vi "Scripting_GetSubVISourcesDrains.vi"(8 "error in (no error)":errorcluster, 11 "SubVIIn":refnum<vi>) -> (0 "error out":errorcluster, 1 "DrainsSources":T1(array[cluster]), 2 "SourceDrains":T2(array[cluster]), 3 "SubVIOut":refnum<vi>)   [LabVIEW 2016]
panel:
  in  "DeleteWiresToSorcesAndDrains(True)":bool=TRUE
  in  "IgnoreCornerTerminals(True)":bool=TRUE
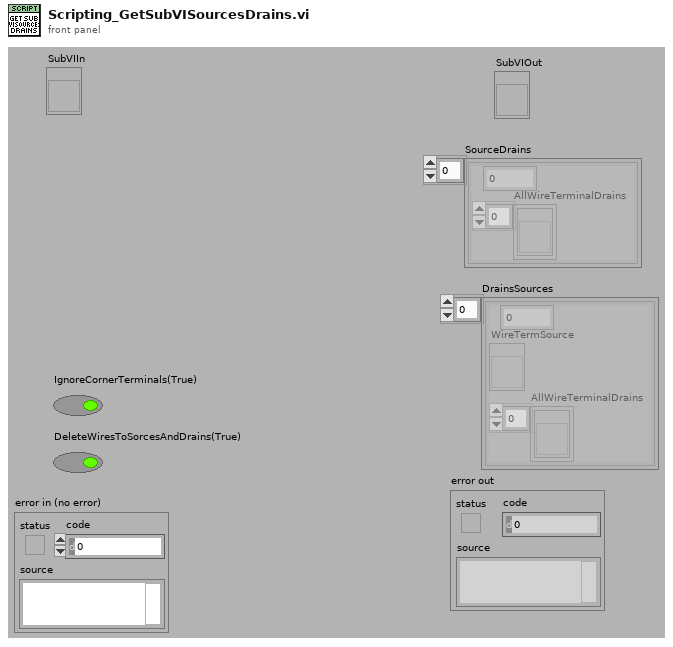
[diagram p1: front panel]
types:
  T1 = cluster{i32, "WireTermSource":refnum<vi>, "AllWireTerminalDrains":refnum<vi>[]}[]
  T2 = cluster{i32, "AllWireTerminalDrains":refnum<vi>[]}[]
  T3 = cluster{i32, "WireTermSource":refnum<vi>, "AllWireTerminalDrains":refnum<vi>[]}
  T4 = cluster{i32, "AllWireTerminalDrains":refnum<vi>[]}
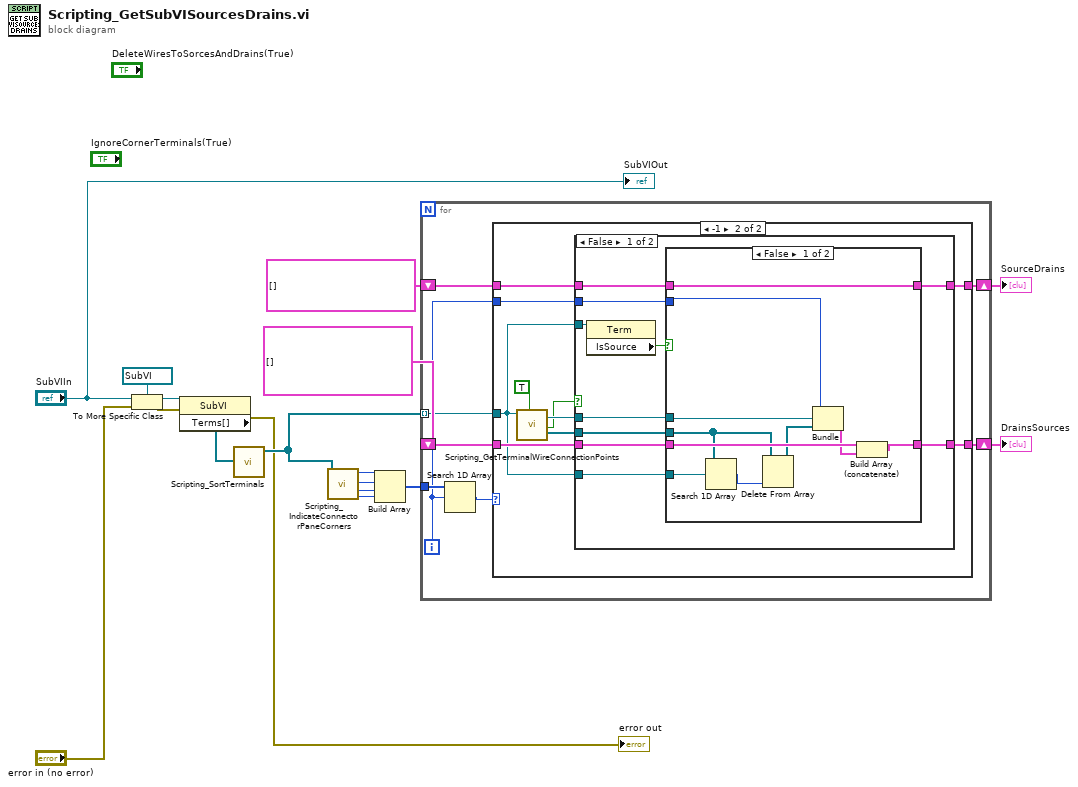
[diagram p0: block diagram]
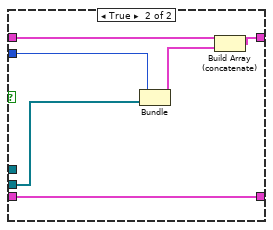
[diagram p3: hidden frame]
diagram:
  n1 = To More Specific Class(target class=refnum<vi> refnum ("Block Diagram"), reference="SubVIIn", error in="error in (no error)") -> (specific class reference=w14:refnum<vi>, error out=w13:errorcluster)
  n2 = property class="SubVI"(reference=w14, error in=w13) -> (error out=→"error out":errorcluster, "Terms[]"=w7:refnum<vi>[])  [unwired: 1 out]
  n3 = call <resource>:"Scripting_SortTerminals.vi"("Terminals[]"=w7) -> ("TerminalsOut[]"=w6:refnum<vi>[])  [unwired: 8 in, 2 out]
  n4 = call <resource>:"Scripting_IndicateConnectorPaneCorners.vi"("Terminals[]"=w6) -> ("RightLower"=w9:i32, "LeftLower"=w10:i32, "RightTop"=w11:i32, "LeftTop"=w12:i32)  [unwired: 7 in]
  n5 = Build Array(w12, w11, w10, w9) -> (w8:i32[])
  n6 = for {
    tunnel: w6 -> [w23] mode=indexing
    tunnel: w8 -> [w25]
    shift-right: [w21] -> w4
    shift-left: T2 [] -> [w22]
    shift-right: [w19] -> w2
    shift-left: T1 [] -> [w20]
    i -> [w18]
    n7 = Search 1D Array(1D array=w25, element=w18) -> (index of element=w24:i32)  [unwired: 1 in]
    n8 = case shown="-1" w24 {
      tunnel: w23 -> [_ w28]
      tunnel: w22 -> [w27 w36]
      tunnel: [w27 w34] -> w21
      tunnel: w20 -> [w26 w33]
      tunnel: [w26 w32] -> w19
      tunnel: w18 -> [_ w29]
      frame 0, Default {
      }
      frame -1 {
        n9 = call <resource>:"Scripting_GetTerminalWireConnectionPoints.vi"("Term Refnum In"=w28, "RemoveWire(False)"=TRUE) -> ("WireTermSource"=w31:refnum<vi>, "NoWireConnected"=w30:bool, "AllWireTerminalDrains"=w35:refnum<vi>[])  [unwired: 9 in, 6 out]
        n10 = case shown="False" w30 {
          tunnel: w28 -> [w47 _]
          tunnel: w36 -> [w45 w65]
          tunnel: w35 -> [w44 _]
          tunnel: [w43 w65] -> w34
          tunnel: w33 -> [w42 w64]
          tunnel: [w41 w64] -> w32
          tunnel: w31 -> [w40 _]
          tunnel: w29 -> [w39 _]
          tunnel: w28 -> [w38 _]
          frame False {
            n11 = property class="Term"(reference=w47) -> ("IsSource"=w46:bool)  [unwired: 1 in, 2 out]
            n12 = case shown="False" w46 {
              tunnel: w45 -> [w57 w62]
              tunnel: w44 -> [w50 w63]
              tunnel: [w57 w60] -> w43
              tunnel: w42 -> [w56 w59]
              tunnel: [w55 w59] -> w41
              tunnel: w40 -> [w53 _]
              tunnel: w39 -> [w54 w58]
              tunnel: w38 -> [w51 _]
              frame False {
                n13 = Search 1D Array(1D array=w50, element=w51) -> (index of element=w49:i32)  [unwired: 1 in]
                n14 = Delete From Array(array=w50, index=w49) -> (array with subset deleted=w48:refnum<vi>[])  [unwired: 1 in, 1 out]
                n15 = Bundle(w54, "WireTermSource"=w53, "AllWireTerminalDrains"=w48) -> (w52:T3)  [unwired: 1 in]
                n16 = Build Array (concatenate)(w56, w52) -> (w55:T1)
              }
              frame True {
                n17 = Bundle(w58, "AllWireTerminalDrains"=w63) -> (w61:T4)  [unwired: 1 in]
                n18 = Build Array (concatenate)(w62, w61) -> (w60:T2)
              }
            }
          }
          frame True {
          }
        }
      }
    }
  }
  "SourceDrains" <- w4
  "DrainsSources" <- w2
  "SubVIOut" <- "SubVIIn"
